vi "kalman-test.vi"() -> ()   [LabVIEW 2014]
uses:
  <vilib>/Platform/TimedLoop/XDataNode/timing_clust.ctl
  <vilib>/Platform/TimedLoop/XDataNode/nitl_modes.ctl
  <vilib>/Platform/TimedLoop/XDataNode/wakeup.ctl
  <vilib>/Analysis/Matrix/Datatypes/RealMatrix.ctl
  <vilib>/platform/TimedLoop/XDataNode/XDataNode.xnode
  <vilib>/Analysis/Matrix/NI_Matrix.lvlib
  <vilib>/ptbypt/NI_PtbyPt.lvlib
  <vilib>/Platform/TimedLoop/XDataNode/XDNodeRunTimeDep.lvlib
panel:
  out "Waveform Chart":cluster{"Real Matrix Element":dbl, dbl}(graph)
  in  "stop":bool
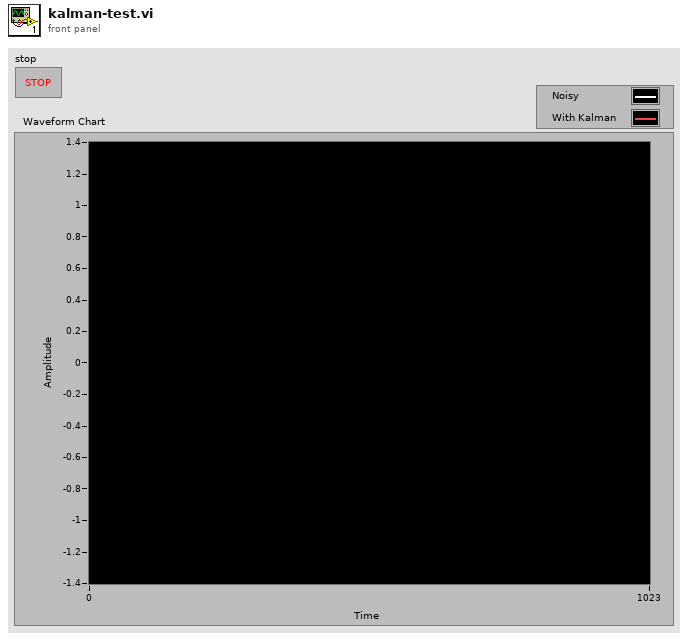
[diagram p1: front panel]
types:
  T1 = typedef "XDNodeRunTimeDep.lvlib/timing_clust.ctl" = cluster{"Expected End [f-1]":u64, "Actual End [f-1]":u64, "Finished Late? [f-1]":bool, "Expected End [i-1]":u64, "Actual End [i-1]":u64, "Finished Late? [i-1]":bool, "Expected Start [i]":u64, "Actual Start [i]":u64, "Expected Start [f]":u64, "Actual Start [f]":u64, "Source Name":string, "Structure Name":string, "Period":i64, "Deadline":i64, "Offset":i64, "Start":i64, "Priority":i32, "Timeout":i32, "Mode":T2, "Wakeup Reason":T3, "Error":errorcluster, "Source Type":string, "Secondary Source Type":string, "Global End Time":u64, "Global Start Time":u64, "Frame Duration":u64, "Iteration Duration":u64, "Assigned CPU":i32, "I/O Scan Engine Mode":u32}
  T2 = typedef "XDNodeRunTimeDep.lvlib/nitl_modes.ctl" = enum32{"No Change", "Process missed periods, maintain original phase", "Discard missed periods, maintain original phase", "Process missed periods, ignore original phase", "Discard missed periods, ignore original phase"}
  T3 = typedef "XDNodeRunTimeDep.lvlib/wakeup.ctl" = enum32{"Normal", "Aborted", "Asynchronous wakeup", "Timing source error", "Timed loop error", "Timeout"}
  T4 = typedef "NI_Matrix.lvlib/RealMatrix.ctl" = dbl[][]
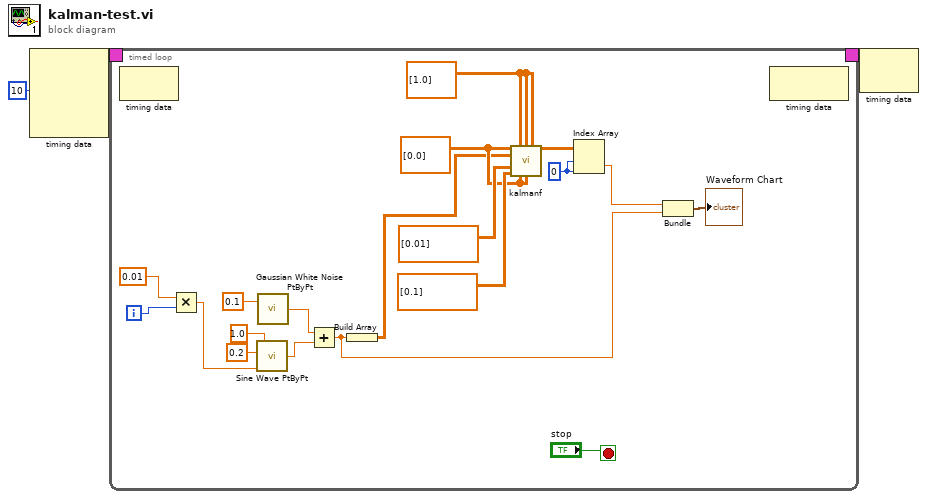
[diagram p0: block diagram]
diagram:
  n1 = node-c288(i64 10 ("Period")) -> (w3:T1)  [unwired: 3 in]
  n2 = timed-loop {
    timing: w3 -> [_]
    timing-out: [_] -> w2
    i -> [w16]
    stop <- "stop" stop-if-true
    w8 = 0 ("index (row)")
    w18 = T4 [[0.0]] ("U")
    w22 = T4 [[1.0]] ("A")
    n3 = node-c288() -> ()  [unwired: 1 in, 1 out]
    n4 = Multiply(x=0.01, y=w16) -> (x*y=w15:dbl)
    n5 = call <vilib>:"Sine Wave PtByPt.vi"("time"=w15, "frequency"=0.2, "amplitude"=1.0) -> ("sine wave"=w12:dbl)  [unwired: 1 in]
    n6 = call <vilib>:"Gaussian White Noise PtByPt.vi"("standard deviation"=0.1) -> ("Gaussian white noise"=w13:dbl)  [unwired: 2 in]
    n7 = Add(x=w13, y=w12) -> (x+y=w6:dbl)
    n8 = Build Array(w6) -> (w11:T4)
    n9 = call "kalmanf.vi"("U"=w18, "A"=w22, "B"=w22, "C"=w22, "y"=w11, "Q"=T4 [[0.01]], "R"=T4 [[0.1]] ("Q"), "xhat0"=w18, "P0"=w18) -> ("xhat"=w4:T4)  [unwired: 6 in]
    n10 = Index Array(array=w4, index (row)=w8, index (col)=w8) -> (element=w7:dbl)
    n11 = Bundle("Real Matrix Element"=w7, w6) -> (→"Waveform Chart":cluster{"Real Matrix Element":dbl, dbl})  [unwired: 1 in]
    n12 = node-c288() -> ()  [unwired: 1 in, 1 out]
  }
  n13 = node-c288(w2) -> ()  [unwired: 1 out]
